vi "calcZslice.vi"(2 "current slice":i32, 3 "# of Slices":u32, 4 "Z-Start (um)":dbl, 5 "Z-end (um)":dbl) -> (0 "zpos (V)":dbl, 1 "zpos (um)":dbl)   [LabVIEW 2015]
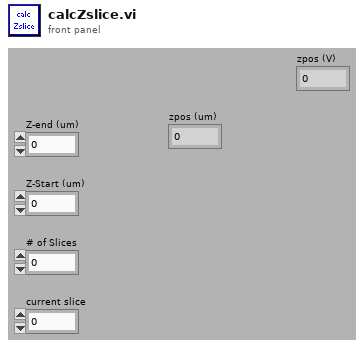
[diagram p1: front panel]
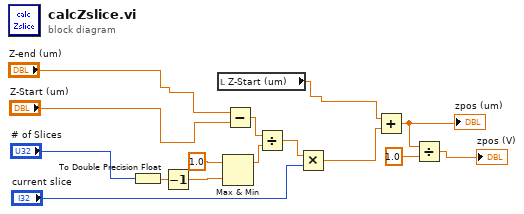
[diagram p0: block diagram]
diagram:
  n1 = To Double Precision Float(number="# of Slices") -> (double precision float=w12:dbl)
  n2 = Decrement(x=w12) -> (x-1=w7:dbl)
  n3 = local read "Z-Start (um)"() -> (w4:dbl)
  n4 = Max & Min(x=1.0 ("y"), y=w7) -> (max(x,y)=w10:dbl)  [unwired: 1 out]
  n5 = Subtract(x="Z-end (um)", y="Z-Start (um)") -> (x-y=w11:dbl)
  n6 = Divide(x=w11, y=w10) -> (x/y=w9:dbl)
  n7 = Multiply(x=w9, y="current slice") -> (x*y=w14:dbl)
  n8 = Add(x=w4, y=w14) -> (x+y=w1:dbl)
  "zpos (um)" <- w1
  n9 = Divide(x=w1, y=1.0) -> (x/y=→"zpos (V)":dbl)
